vi "Set Title.vi"(8 "error in (no error)":errorcluster, 11 "[V] Waveform in":refnum<class "[V] Waveform.lvclass">) -> (0 "error out":errorcluster, 3 "[V] Waveform out":refnum<class "[V] Waveform.lvclass">)   [LabVIEW 2020, in "[V] Waveform.lvlib" / "[V] Waveform.lvclass"]
uses:
  [V] Waveform.lvclass
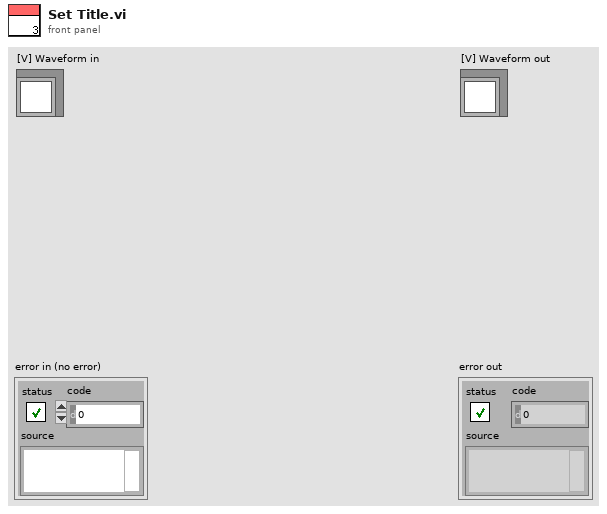
[diagram p1: front panel]
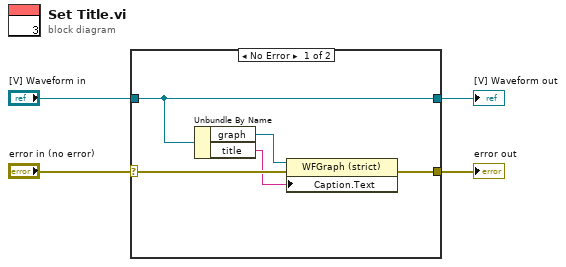
[diagram p0: block diagram]
diagram:
  n1 = case shown="No Error" "error in (no error)" {
    selector: "error in (no error)" -> [w8 w11]
    tunnel: [w6 w11] -> w3
    tunnel: [w9 w10] -> w1
    tunnel: "[V] Waveform in" -> [w9 w10]
    frame No Error {
      n2 = Unbundle By Name(w9) -> ("graph"=w7:refnum<vi>, "title"=w5:string)
      n3 = property class="WFGraph (strict)"(reference=w7, error in=w8, "Caption.Text"=w5) -> (error out=w6:errorcluster)  [unwired: 1 out]
    }
    frame Error {
    }
  }
  "error out" <- w3
  "[V] Waveform out" <- w1
